vi "Obtain Pref Group.vi"(8 "error in (no error)":errorcluster, 10 "Group":string, 11 "PrefsDB in":refnum<class "PrefsDB.lvclass">) -> (0 "error out":errorcluster, 2 "Pref Group":refnum<class "Pref Group.lvclass">, 3 "PrefsDB out":refnum<class "PrefsDB.lvclass">)   [LabVIEW 2020, in "User Prefs.lvlib" / "PrefsDB.lvclass"]
uses:
  PrefsDB.lvclass
  PrefsDB.lvclass/PrefsDB.ctl
  Pref Group/Pref Group.lvclass
  lv-cdm/CDM-Config/Config Manager/Config Manager.lvclass
  Pref Group.ctl
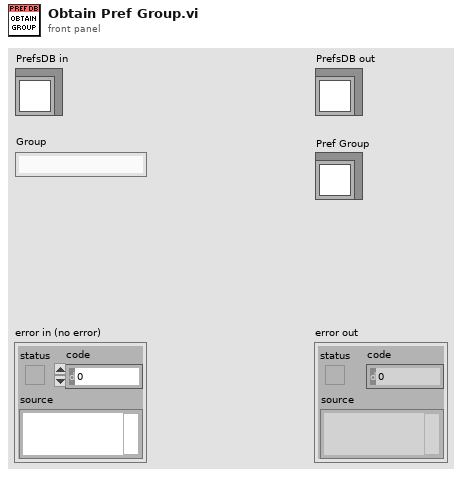
[diagram p1: front panel]
types:
  T1 = typedef "User Prefs.lvlib/PrefsDB.lvclass/Pref Group.ctl" = cluster{"Config Manager":refnum<class "Config Manager.lvclass">, "Group":string}
  T2 = typedef "User Prefs.lvlib/PrefsDB.lvclass/Ref Data.ctl" = cluster{"Map":map{string, T1}}
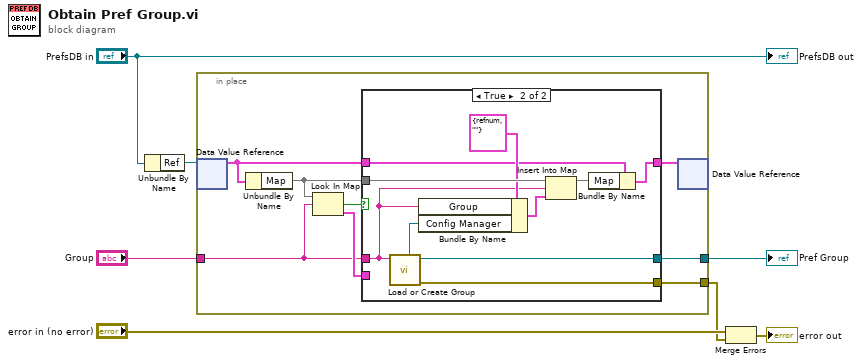
[diagram p0: block diagram]
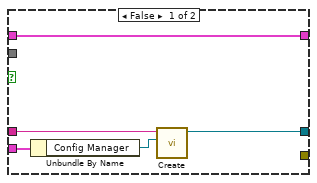
[diagram p2: hidden frame]
diagram:
  n1 = Unbundle By Name("PrefsDB in") -> ("Ref"=w5:refnum<data-value>)
  n2 = in-place {
    in-place-border: "Group" -> [w13]
    in-place-border: [w12] -> w3
    in-place-border: [w8] -> w1
    n3 = in-place-dvr #1(w5) -> (w10:T2)  [unwired: 1 out]
    n4 = Unbundle By Name(w10) -> ("Map"=w9:map{string, T1})
    n5 = Look In Map(map=w9, key=w13) -> (key not found?=w15:bool, value=w14:T1)  [unwired: 1 in]
    n6 = case shown="True" w15 {
      tunnel: w14 -> [w20 _]
      tunnel: w13 -> [w19 w24]
      tunnel: [w17 w22] -> w12
      tunnel: [w16 w25] -> w11
      tunnel: w10 -> [w16 w27]
      tunnel: w9 -> [_ w30]
      tunnel: [_ w21] -> w8
      frame False {
        n7 = Unbundle By Name(w20) -> ("Config Manager"=w18:refnum<class "Config Manager.lvclass">)
        n8 = call "Create.vi"("Config Manager"=w18, "Group"=w19) -> ("Pref Group out"=w17:refnum<class "Pref Group.lvclass">)  [unwired: 8 in, 1 out]
      }
      frame True {
        n9 = call "Load or Create Group.vi"("Group Name"=w24) -> ("error out"=w21:errorcluster, "Pref Group"=w22:refnum<class "Pref Group.lvclass">, "Config Manager"=w23:refnum<class "Config Manager.lvclass">)  [unwired: 8 in]
        n10 = Bundle By Name(cluster=T1 {"Config Manager"=refnum, "Group"=""} ("value"), "Group"=w24, "Config Manager"=w23) -> (w28:T1)
        n11 = Insert Into Map(map in=w30, key=w24, value=w28) -> (map out=w26:map{string, T1})  [unwired: 2 out]
        n12 = Bundle By Name(cluster=w27, "Map"=w26) -> (w25:T2)
      }
    }
    n13 = in-place-dvr #1(w11) -> ()  [unwired: 2 out]
  }
  "Pref Group" <- w3
  n14 = Merge Errors("error in (no error)", w1) -> (→"error out":errorcluster)
  "PrefsDB out" <- "PrefsDB in"
